vi "Panel.vi"(11 "MuxPanel in":refnum<class "MuxPanel.lvclass">) -> ()   [LabVIEW 2022 SP3, in "TouchControl.lvlib" / "MuxPanel.lvclass"]
uses:
  MuxPanel.lvclass
  C:/Program Files (x86)/National Instruments/LabVIEW 2022/vi.lib/IlluminatedG/IG OOPanel/OOPanel/Panel/Panel.lvclass
  MUX Button.ctl
  <vilib>/IlluminatedG/IG OOPanel/OOPanel/Panel/Basic UI State.ctl
  MuxPanel.lvclass/MuxPanel.ctl
  <vilib>/IlluminatedG/IG OOPanel/OOPanel/Panel/Panel.lvclass
  <vilib>/IlluminatedG/IG OOPanel/OOPanel/OOPanel.lvlib
  TouchControl.lvlib
  C:/dev/illuminatedg/TouchControl/TouchControl/MuxPanel/MuxPanel.lvclass
panel:
  in  "Desktop Bench":bool
  in  "Work Dock Bench":bool
  in  "Work Dock Main":bool
  in  "Desktop Main":bool
  in  "Input 16":bool
  in  "Input 15":bool
  in  "Input 14":bool
  in  "Input 13":bool
  in  "Input 12":bool
  in  "Input 11":bool
  in  "Input 10":bool
  in  "Input 9":bool
  in  "MUX Button 16":T1
  in  "MUX Button 15":T1
  in  "MUX Button 14":T1
  in  "MUX Button 13":T1
  in  "MUX Button 12":T1
  in  "MUX Button 11":T1
  in  "MUX Button 10":T1
  in  "MUX Button 9":T1
  in  "Input 8":bool
  in  "Input 7":bool
  in  "Input 6":bool
  in  "Input 5":bool
  in  "Input 4":bool
  in  "Input 3":bool
  in  "Input 2":bool
  in  "Input 1":bool
  in  "MUX Button 8":T1
  in  "MUX Button 7":T1
  in  "MUX Button 6":T1
  in  "MUX Button 5":T1
  in  "MUX Button 4":T1
  in  "MUX Button 3":T1
  in  "MUX Button 2":T1
  in  "MUX Button 1":T1
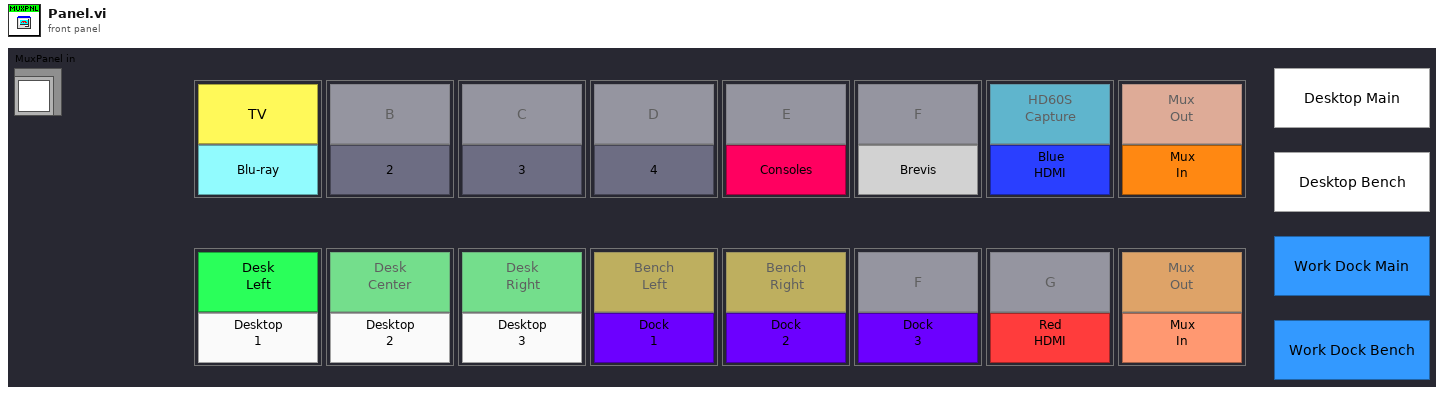
[diagram p1: front panel]
types:
  T1 = typedef "TouchControl.lvlib/MuxPanel.lvclass/MUX Button.ctl" = cluster{"A":bool, "Input":string}
  T2 = typedef "OOPanel.lvlib/Panel.lvclass/Basic UI State.ctl" = enum16{"Init", "Run", "Close"}
  T3 = typedef "TouchControl.lvlib/MUX Config.ctl" = cluster{"Outputs":T4[], "Inputs":T4[]}
  T4 = typedef "TouchControl.lvlib/MUX Element.ctl" = cluster{string, u32}
  T5 = enum8{"Enabled", "Disabled", "Disabled and Grayed Out"}
  T6 = typedef "TouchControl.lvlib/MuxPanel.lvclass/Events.ctl" = cluster{"Delay":refnum<user-event>, "Connect":refnum<user-event>}
  T7 = typedef "OOPanel.lvlib/Panel.lvclass/Panel Events.ctl" = cluster{"Visbility":refnum<user-event>, "Close":refnum<user-event>}
  T8 = typedef "TouchControl.lvlib/MUX Selection.ctl" = enum16{"Computers", "Others"}
  T9 = typedef "OOPanel.lvlib/Visibility State.ctl" = enum16{"Idle", "Closed", "Hidden", "Visible", "Subpanel", "Hidden Subpanel"}
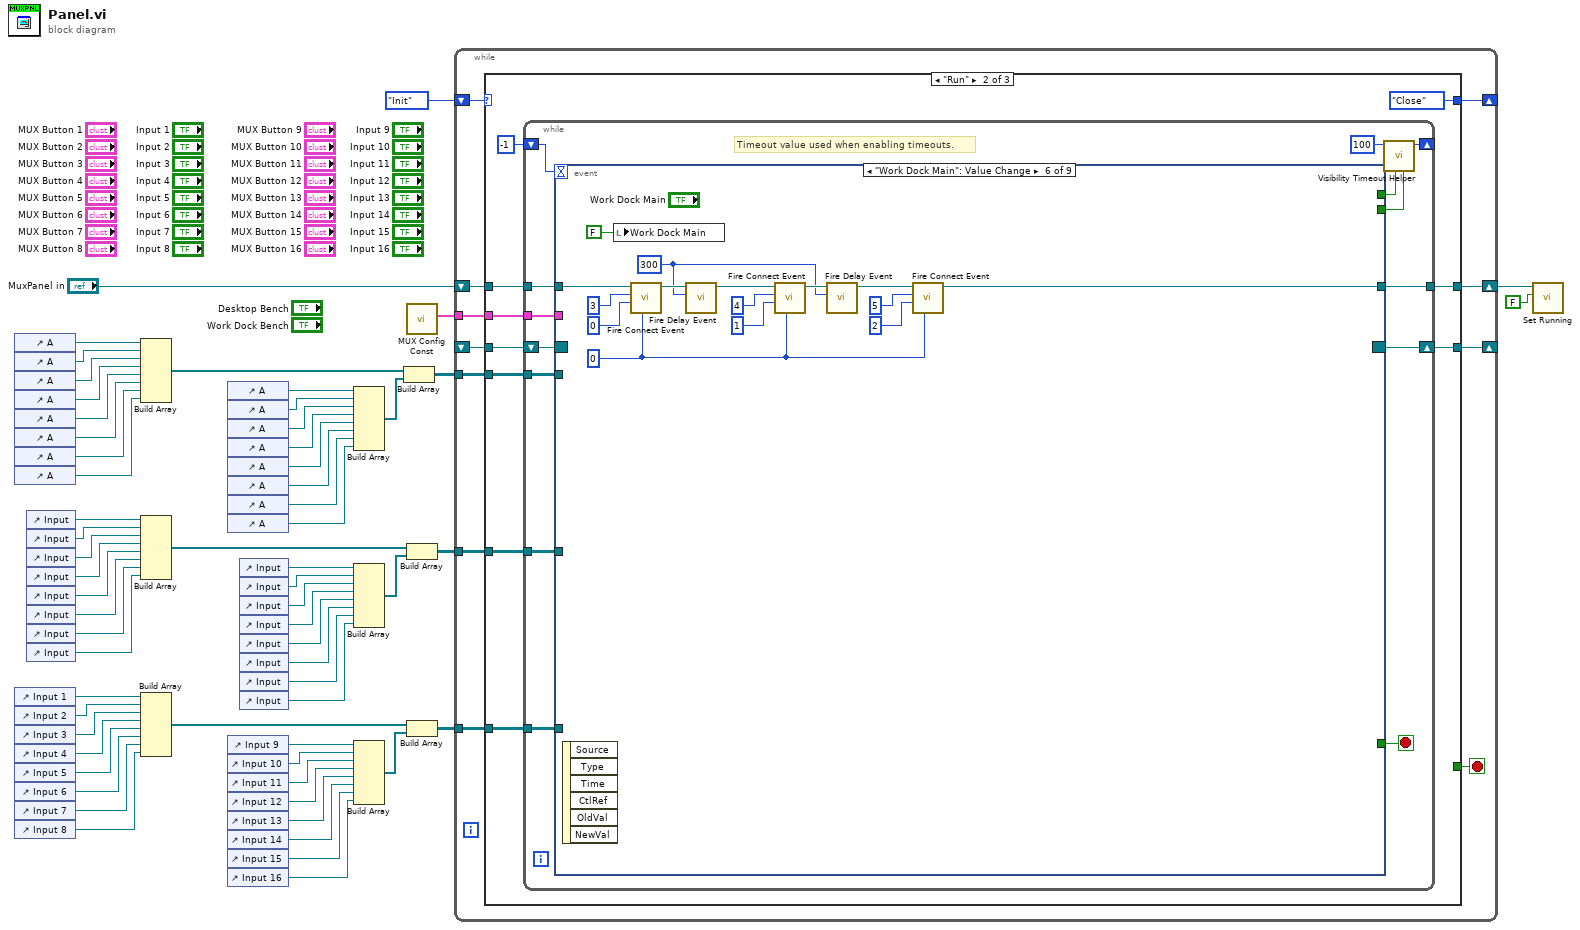
[diagram p0: block diagram]
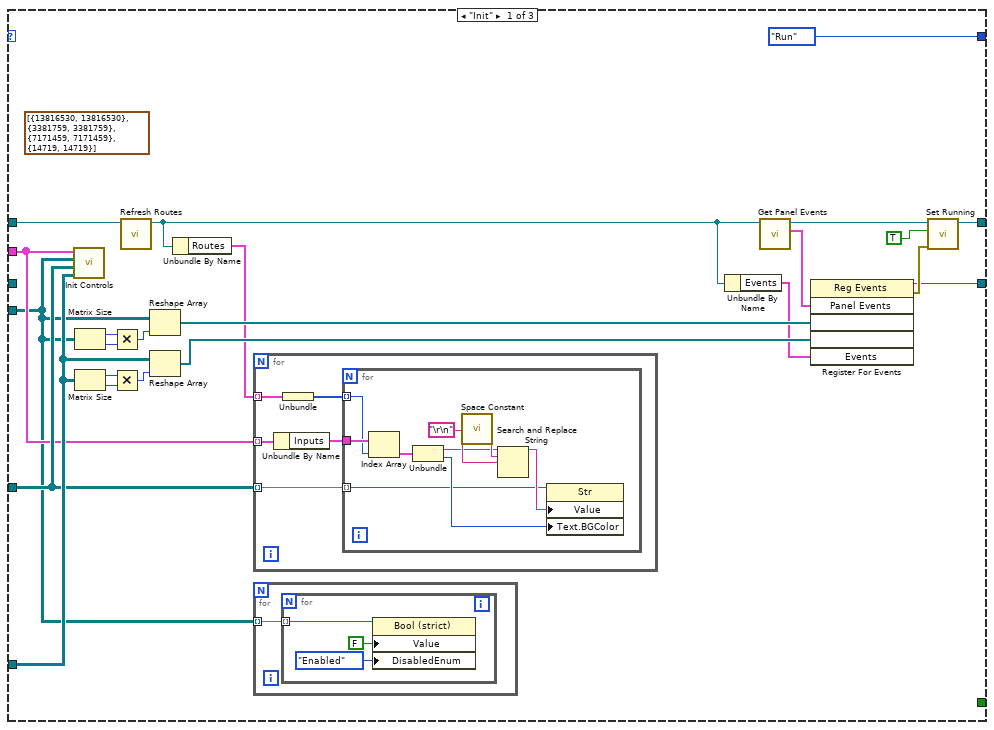
[diagram p2: hidden frame]
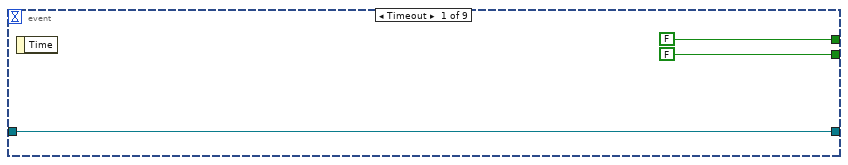
[diagram p3: hidden frame]
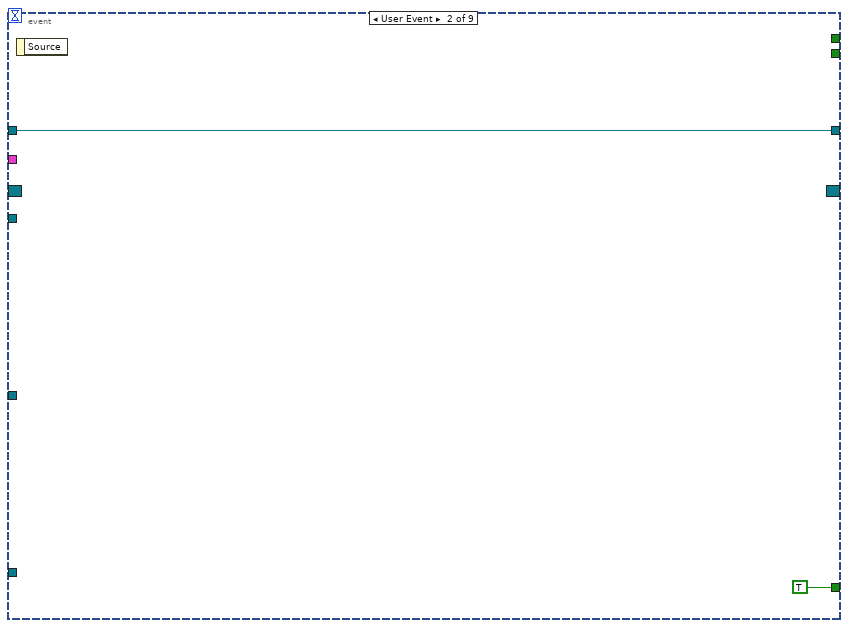
[diagram p4: hidden frame]
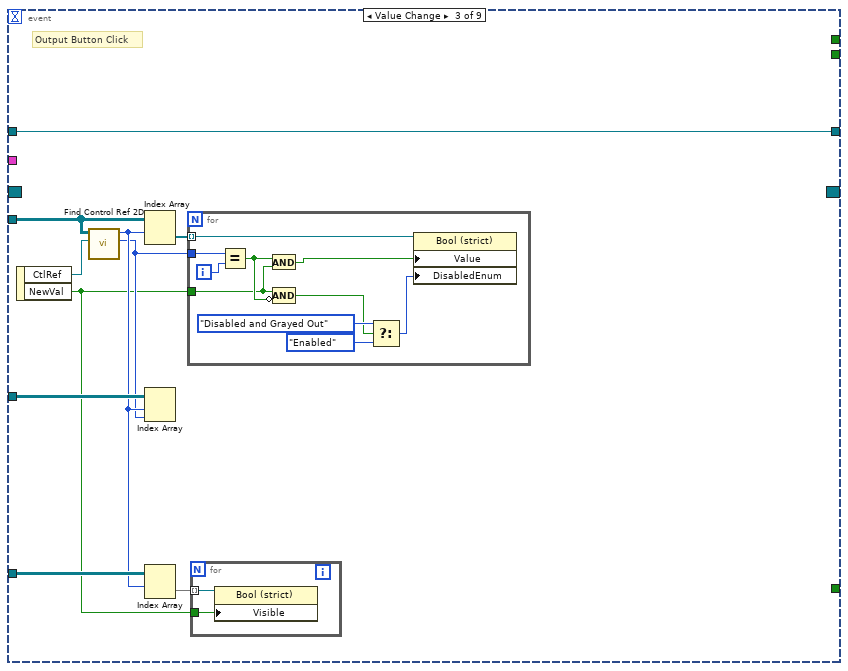
[diagram p5: hidden frame]
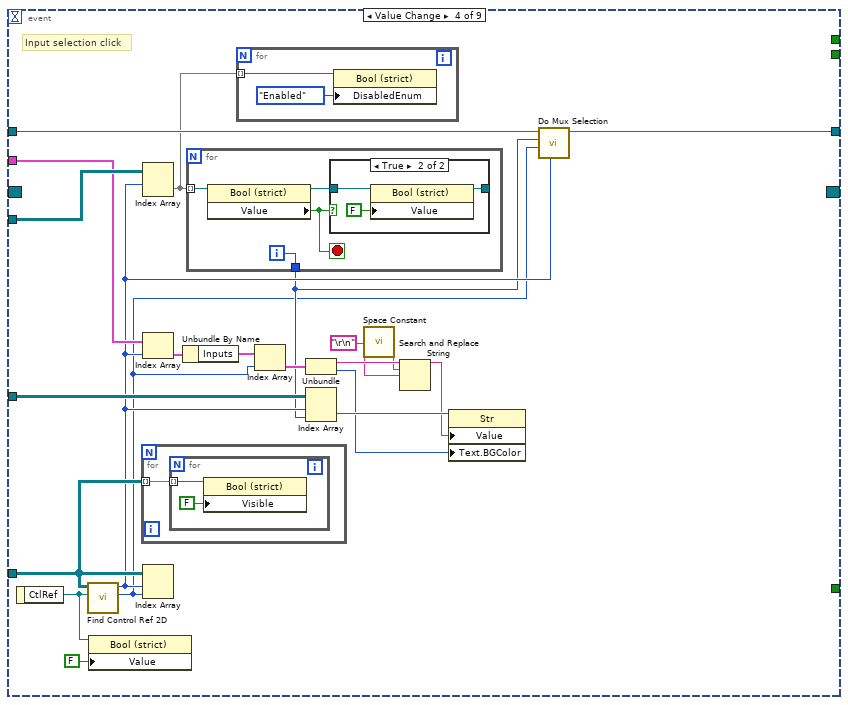
[diagram p6: hidden frame]
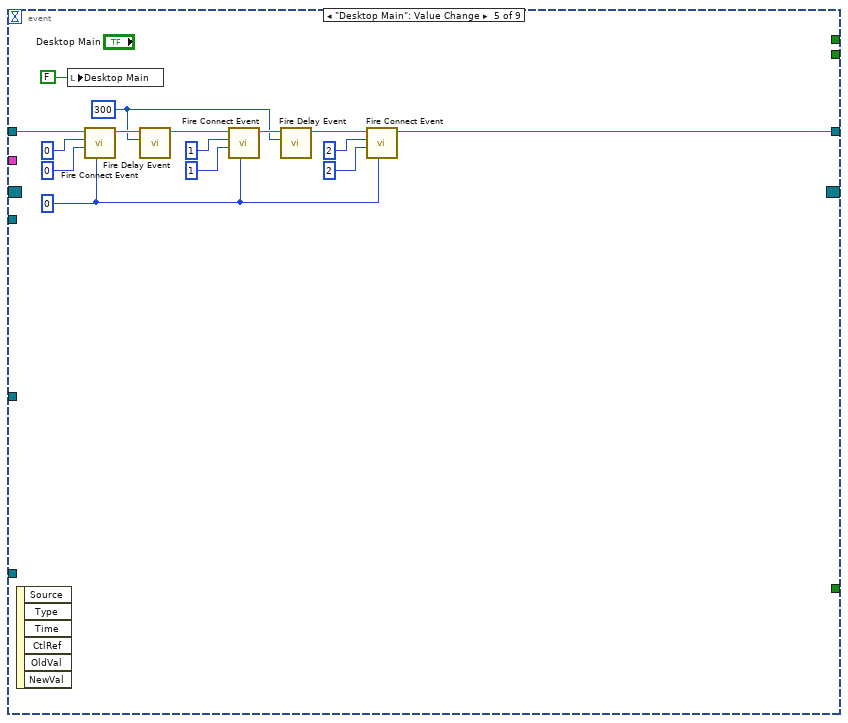
[diagram p8: hidden frame]
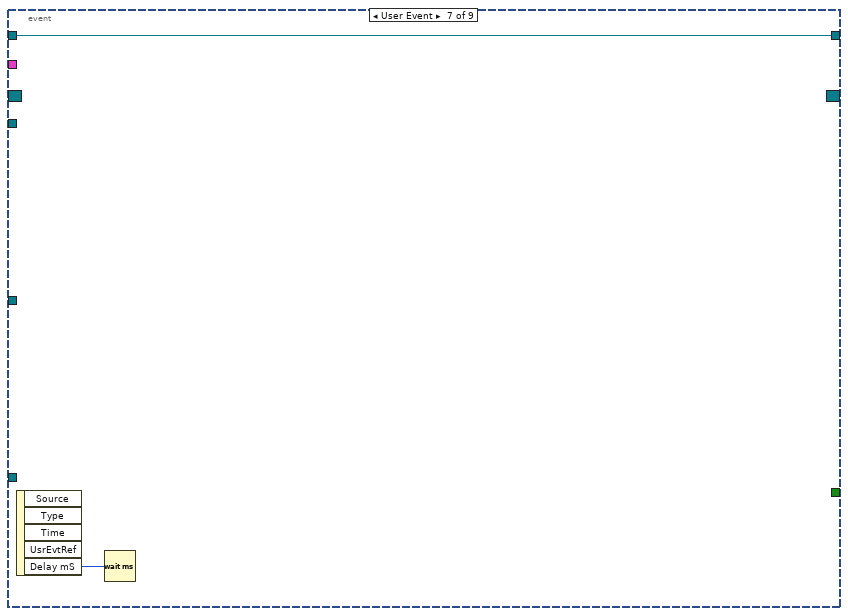
[diagram p9: hidden frame]
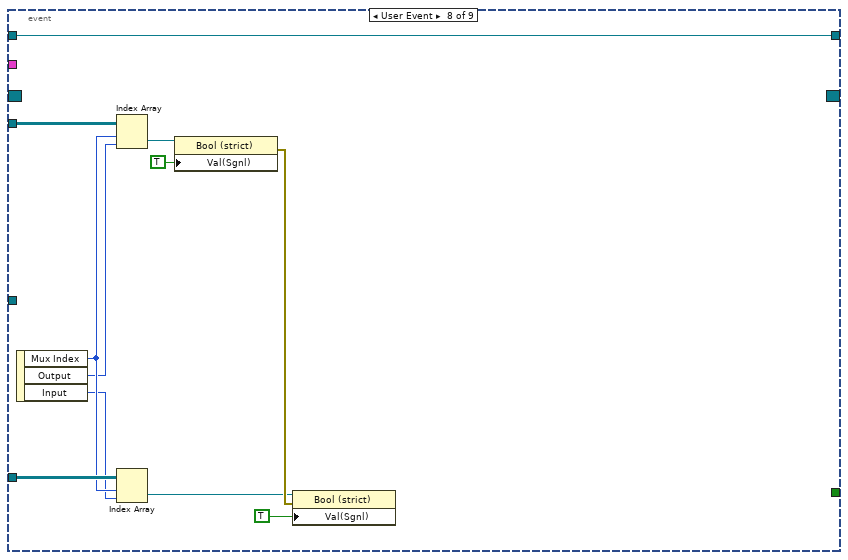
[diagram p10: hidden frame]
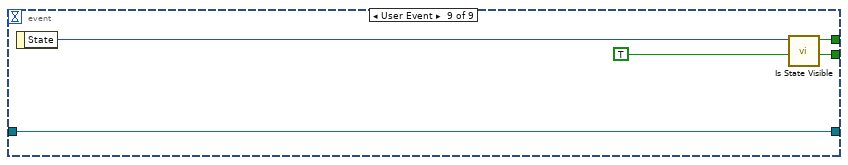
[diagram p11: hidden frame]
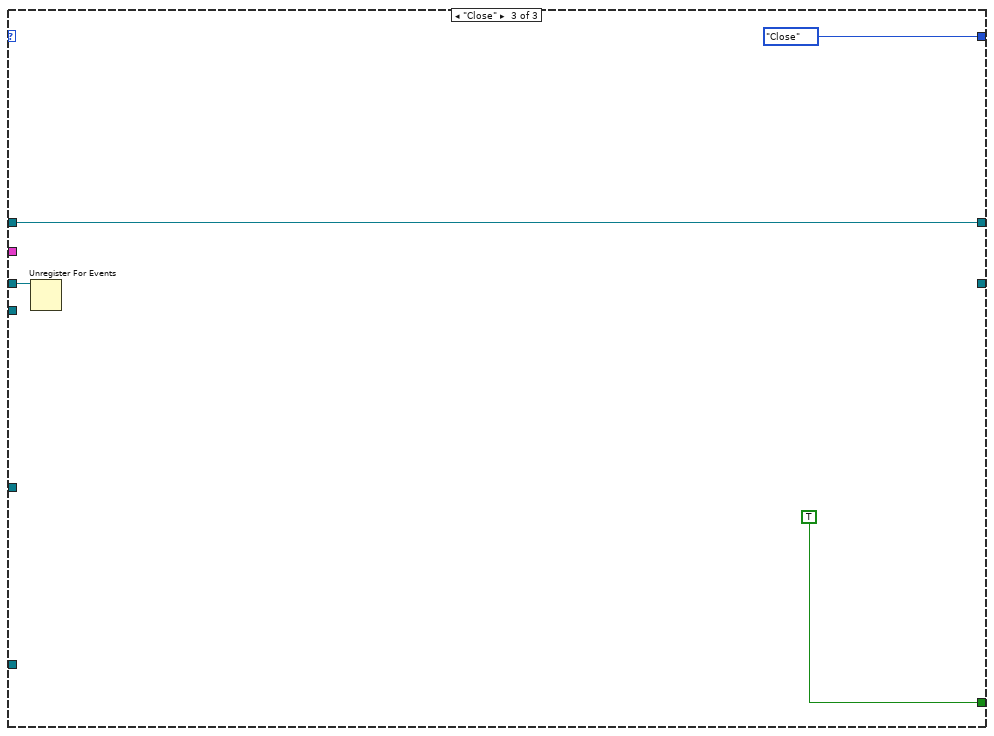
[diagram p12: hidden frame]
diagram:
  n1 = control-ref of="A"() -> (w58:refnum<vi>)
  n2 = control-ref of="A"() -> (w57:refnum<vi>)
  n3 = control-ref of="A"() -> (w56:refnum<vi>)
  n4 = control-ref of="A"() -> (w55:refnum<vi>)
  n5 = control-ref of="A"() -> (w54:refnum<vi>)
  n6 = control-ref of="A"() -> (w53:refnum<vi>)
  n7 = control-ref of="A"() -> (w52:refnum<vi>)
  n8 = control-ref of="A"() -> (w51:refnum<vi>)
  n9 = control-ref of="Input 1"() -> (w49:refnum<vi>)
  n10 = control-ref of="Input 2"() -> (w48:refnum<vi>)
  n11 = control-ref of="Input 3"() -> (w47:refnum<vi>)
  n12 = control-ref of="Input 4"() -> (w46:refnum<vi>)
  n13 = control-ref of="Input 5"() -> (w45:refnum<vi>)
  n14 = control-ref of="Input 6"() -> (w44:refnum<vi>)
  n15 = control-ref of="Input 7"() -> (w43:refnum<vi>)
  n16 = control-ref of="Input 8"() -> (w42:refnum<vi>)
  n17 = control-ref of="Input"() -> (w50:refnum<vi>)
  n18 = control-ref of="Input"() -> (w40:refnum<vi>)
  n19 = control-ref of="Input"() -> (w39:refnum<vi>)
  n20 = control-ref of="Input"() -> (w38:refnum<vi>)
  n21 = control-ref of="Input"() -> (w37:refnum<vi>)
  n22 = control-ref of="Input"() -> (w36:refnum<vi>)
  n23 = control-ref of="Input"() -> (w35:refnum<vi>)
  n24 = control-ref of="Input"() -> (w41:refnum<vi>)
  n25 = Build Array(w58, w57, w56, w55, w54, w53, w52, w51) -> (w34:refnum<vi>[])
  n26 = Build Array(w50, w40, w39, w38, w37, w36, w35, w41) -> (w33:refnum<vi>[])
  n27 = Build Array(w49, w48, w47, w46, w45, w44, w43, w42) -> (w32:refnum<vi>[])
  n28 = control-ref of="A"() -> (w8:refnum<vi>)
  n29 = control-ref of="A"() -> (w9:refnum<vi>)
  n30 = control-ref of="A"() -> (w10:refnum<vi>)
  n31 = control-ref of="A"() -> (w11:refnum<vi>)
  n32 = control-ref of="A"() -> (w12:refnum<vi>)
  n33 = control-ref of="A"() -> (w13:refnum<vi>)
  n34 = control-ref of="A"() -> (w14:refnum<vi>)
  n35 = control-ref of="A"() -> (w15:refnum<vi>)
  n36 = control-ref of="Input 9"() -> (w17:refnum<vi>)
  n37 = control-ref of="Input 10"() -> (w18:refnum<vi>)
  n38 = control-ref of="Input 11"() -> (w19:refnum<vi>)
  n39 = control-ref of="Input 12"() -> (w20:refnum<vi>)
  n40 = control-ref of="Input 13"() -> (w21:refnum<vi>)
  n41 = control-ref of="Input 14"() -> (w22:refnum<vi>)
  n42 = control-ref of="Input 15"() -> (w23:refnum<vi>)
  n43 = control-ref of="Input 16"() -> (w24:refnum<vi>)
  n44 = control-ref of="Input"() -> (w16:refnum<vi>)
  n45 = control-ref of="Input"() -> (w26:refnum<vi>)
  n46 = control-ref of="Input"() -> (w27:refnum<vi>)
  n47 = control-ref of="Input"() -> (w28:refnum<vi>)
  n48 = control-ref of="Input"() -> (w29:refnum<vi>)
  n49 = control-ref of="Input"() -> (w30:refnum<vi>)
  n50 = control-ref of="Input"() -> (w31:refnum<vi>)
  n51 = control-ref of="Input"() -> (w25:refnum<vi>)
  n52 = Build Array(w8, w9, w10, w11, w12, w13, w14, w15) -> (w6:refnum<vi>[])
  n53 = Build Array(w16, w26, w27, w28, w29, w30, w31, w25) -> (w4:refnum<vi>[])
  n54 = Build Array(w17, w18, w19, w20, w21, w22, w23, w24) -> (w2:refnum<vi>[])
  n55 = Build Array(w34, w6) -> (w7:refnum<vi>[][])
  n56 = call "MUX Config Const.vi"() -> ("MUX Config"=w1:T3[])  [unwired: 11 in]
  n57 = Build Array(w33, w4) -> (w5:refnum<vi>[][])
  n58 = Build Array(w32, w2) -> (w3:refnum<vi>[][])
  n59 = while {
    shift-right: [w72] -> _
    shift-left: _ -> [w73]
    shift-right: [w70] -> _
    shift-left: Basic_UI_State."Init" ("Basic UI State") -> [w71]
    shift-right: [w68] -> w62
    shift-left: "MuxPanel in" -> [w67]
    tunnel: w7 -> [w66]
    tunnel: w5 -> [w65]
    tunnel: w3 -> [w64]
    tunnel: w1 -> [w63]
    stop <- w69 stop-if-true
    n60 = case shown="\"Run\"" w71 {
      tunnel: w73 -> [_ w124 w248]
      tunnel: [w93 w122 _] -> w72
      tunnel: [Basic_UI_State."Run" ("Basic UI State") Basic_UI_State."Close" ("Basic UI State") Basic_UI_State."Close" ("Basic UI State")] -> w70
      tunnel: [_ _ TRUE] -> w69
      tunnel: [w92 w119 w247] -> w68
      tunnel: w67 -> [w91 w120 w247]
      tunnel: w66 -> [w74 w118 _]
      tunnel: w65 -> [w79 w117 _]
      tunnel: w64 -> [w81 w116 _]
      tunnel: w63 -> [w78 w115 _]
      frame "Init" {
        (unwired) cluster{u32, u32}[] [{13816530, 13816530}, {3381759, 3381759}, {7171459, 7171459}, {14719, 14719}] ("Colors [4]")
        n61 = call "Init Controls.vi"("Inputs"=w81, "Labels"=w79, "Outputs"=w74, "MUX Config"=w78) -> ()  [unwired: 8 in]
        n62 = Matrix Size(0:w74) -> (1:w88:i32, 2:w87:i32)
        n63 = Matrix Size(0:w81) -> (1:w84:i32, 2:w83:i32)
        n64 = Multiply(x=w88, y=w87) -> (x*y=w86:i32)
        n65 = Multiply(x=w84, y=w83) -> (x*y=w82:i32)
        n66 = call "Refresh Routes.vi"("MuxPanel in"=w91) -> ("MuxPanel out"=w76:refnum<class "MuxPanel.lvclass">)  [unwired: 9 in, 1 out]
        n67 = Reshape Array(w74, w86) -> (w85:refnum<vi>[])
        n68 = Reshape Array(w81, w82) -> (w80:refnum<vi>[])
        n69 = Unbundle By Name(w76) -> ("Routes"=w77:cluster{"Mux Route":i32[]}[])
        n70 = for {
          tunnel: w79 -> [w101] mode=indexing
          tunnel: w78 -> [w105] mode=indexing
          tunnel: w77 -> [w104] mode=indexing
          n71 = Unbundle By Name(w105) -> ("Inputs"=w102:T4[])
          n72 = Unbundle(w104) -> ("Mux Route"=w103:i32[])
          n73 = for {
            tunnel: w103 -> [w110] mode=indexing
            tunnel: w102 -> [w111]
            tunnel: w101 -> [w106] mode=indexing
            n74 = Index Array(array=w111, index=w110) -> (element=w109:T4)
            n75 = Unbundle(w109) -> (w108:string, w107:u32)
            n76 = call <vilib>:"Space Constant.vi"() -> ("String"=w114:string)
            n77 = Search and Replace String(input string=w108, search string=w114, replace string="\r\n") -> (result string=w112:string)  [unwired: 5 in, 3 out]
            n78 = property class="Str"(reference=w106, "Value"=w112, "Text.BGColor"=w107) -> ()  [unwired: 1 in, 2 out]
          }
        }
        n79 = for {
          tunnel: w74 -> [w97] mode=indexing
          n80 = for {
            tunnel: w97 -> [w100] mode=indexing
            n81 = property class="Bool (strict)"(reference=w100, "Value"=FALSE, "DisabledEnum"=T5."Enabled" ("Disabled")) -> ()  [unwired: 1 in, 2 out]
          }
        }
        n82 = Unbundle By Name(w76) -> ("Events"=w75:T6)
        n83 = call <vilib>:"Get Panel Events.vi"("Panel in"=w76) -> ("Panel Events"=w89:T7, "Panel out"=w90:refnum<class "MuxPanel.lvclass">)  [unwired: 8 in, 1 out]
        n84 = register-events(w89, w85, w80, w75) -> (reference out=w93:refnum<event-registration>, error out=w95:errorcluster)  [unwired: 2 in]
        n85 = call <vilib>:"Set Running.vi"("error in (no error)"=w95, "Running"=TRUE, "Panel in"=w90) -> ("Panel out"=w92:refnum<class "MuxPanel.lvclass">)  [unwired: 7 in, 1 out]
      }
      frame "Run" {
        n86 = while {
          shift-right: [w134] -> w122
          shift-left: w124 -> [w135]
          shift-right: [w137] -> _
          shift-left: -1 ("Timeout") -> [w136]
          tunnel: w120 -> [w130]
          tunnel: [w129] -> w119
          tunnel: w118 -> [w128]
          tunnel: w117 -> [w127]
          tunnel: w116 -> [w126]
          tunnel: w115 -> [w125]
          stop <- w131 stop-if-true
          # "Timeout value used when enabling timeouts."
          n87 = event shown="[5] \"Work Dock Main\": Value Change" {
            selector: w135 -> [_ _ _ _ _ _ _ _ _]
            dyn-events: [_ _ _ _ _ _ _ _ _] -> w134
            timeout: w136 -> [_ _ _ _ _ _ _ _ _]
            tunnel: [FALSE _ _ _ _ _ _ _ w245] -> w133
            tunnel: [FALSE _ _ _ _ _ _ _ TRUE] -> w132
            tunnel: [_ TRUE _ _ _ _ _ _ _] -> w131
            tunnel: w130 -> [w139 w142 w153 w185 w214 w229 w231 w241 w243]
            tunnel: [w139 w142 w153 w169 w200 w215 w231 w241 w243] -> w129
            tunnel: w128 -> [_ _ w151 w184 _ _ _ w240 _]
            tunnel: w127 -> [_ _ w150 w183 _ _ _ _ _]
            tunnel: w126 -> [_ _ w149 w182 _ _ _ w239 _]
            tunnel: w125 -> [_ _ _ w181 _ _ _ _ _]
            event Timeout {
              n88 = event-data() -> ()  [unwired: 1 in, 1 out]
            }
            event User Event {
              n89 = event-data() -> ()  [unwired: 1 in, 1 out]
            }
            event Value Change {
              # "Output Button Click"
              n90 = event-data() -> ("CtlRef"=w152:refnum<vi>, "NewVal"=w144:bool)  [unwired: 1 in]
              n91 = call "Find Control Ref 2D.vi"("Ctl Refnum"=w152, "2D Array"=w151) -> ("Index"=w145:i32, "MUX Selection"=w148:T8)  [unwired: 8 in]
              n92 = Index Array(array=w151, index (row)=w148) -> (element=w146:refnum<vi>[])  [unwired: 1 in]
              n93 = Index Array(array=w150, index (row)=w148, index (col)=w145) -> ()  [unwired: 1 out]
              n94 = Index Array(array=w149, index (row)=w148) -> (element=w147:refnum<vi>[])  [unwired: 1 in]
              n95 = for {
                tunnel: w146 -> [w163] mode=indexing
                tunnel: w145 -> [w162]
                tunnel: w144 -> [w155]
                i -> [w157]
                n96 = Equal?(x=w162, y=w157) -> (x = y?=w156:bool)
                n97 = And(x=w156, y=w155) -> (x .and. y?=w161:bool)
                n98 = Compound Arithmetic op=AND(w155, invert w156) -> (w154:bool)
                n99 = Select(t=T5."Disabled and Grayed Out" ("Disabled"), s=w154, f=T5."Enabled" ("Disabled")) -> (s? t:f=w158:T5)
                n100 = property class="Bool (strict)"(reference=w163, "Value"=w161, "DisabledEnum"=w158) -> ()  [unwired: 1 in, 2 out]
              }
              n101 = for {
                tunnel: w147 -> [w165] mode=indexing
                tunnel: w144 -> [w164]
                n102 = property class="Bool (strict)"(reference=w165, "Visible"=w164) -> ()  [unwired: 1 in, 2 out]
              }
            }
            event Value Change {
              # "Input selection click"
              n103 = event-data() -> ("CtlRef"=w177:refnum<vi>)  [unwired: 1 in]
              n104 = call "Find Control Ref 2D.vi"("Ctl Refnum"=w177, "2D Array"=w182) -> ("Index"=w166:i32, "MUX Selection"=w168:T8)  [unwired: 8 in]
              n105 = property class="Bool (strict)"(reference=w177, "Value"=FALSE) -> ()  [unwired: 1 in, 2 out]
              n106 = for {
                tunnel: w182 -> [w197] mode=indexing
                n107 = for {
                  tunnel: w197 -> [w199] mode=indexing
                  n108 = property class="Bool (strict)"(reference=w199, "Visible"=FALSE) -> ()  [unwired: 1 in, 2 out]
                }
              }
              n109 = Index Array(array=w184, index (row)=w168) -> (element=w170:refnum<vi>[])  [unwired: 1 in]
              n110 = Index Array(array=w181, index=w168) -> (element=w180:T3)
              n111 = Index Array(array=w182, index (row)=w168, index (col)=w166) -> ()  [unwired: 1 out]
              n112 = Unbundle By Name(w180) -> ("Inputs"=w179:T4[])
              n113 = for {
                tunnel: w170 -> [w192] mode=indexing
                tunnel: [w189] -> w167
                i -> [w189]
                stop <- w190 stop-if-true
                n114 = property class="Bool (strict)"(reference=w192) -> (reference out=w191:refnum<vi>, "Value"=w190:bool)  [unwired: 1 in, 1 out]
                n115 = case shown="True" w190 {
                  tunnel: w191 -> [w193 w196]
                  tunnel: [w193 w194] -> _
                  frame False {
                  }
                  frame True {
                    n116 = property class="Bool (strict)"(reference=w196, "Value"=FALSE) -> (reference out=w194:refnum<vi>)  [unwired: 1 in, 1 out]
                  }
                }
              }
              n117 = for {
                tunnel: w170 -> [w187] mode=indexing
                n118 = property class="Bool (strict)"(reference=w187, "DisabledEnum"=T5."Enabled" ("Disabled")) -> ()  [unwired: 1 in, 2 out]
              }
              n119 = Index Array(array=w179, index=w166) -> (element=w178:T4)
              n120 = Unbundle(w178) -> (w186:string, w174:u32)
              n121 = Index Array(array=w183, index (row)=w168, index (col)=w167) -> (element=w175:refnum<vi>)
              n122 = call <vilib>:"Space Constant.vi"() -> ("String"=w173:string)
              n123 = Search and Replace String(input string=w186, search string=w173, replace string="\r\n") -> (result string=w171:string)  [unwired: 5 in, 3 out]
              n124 = property class="Str"(reference=w175, "Value"=w171, "Text.BGColor"=w174) -> ()  [unwired: 1 in, 2 out]
              n125 = call "Do Mux Selection.vi"("MUX Selection"=w168, "Input Index"=w166, "Output Index"=w167, "MuxPanel in"=w185) -> ("MuxPanel out"=w169:refnum<class "MuxPanel.lvclass">)  [unwired: 6 in, 1 out]
            }
            event "Desktop Main": Value Change {
              w205 = 300 ("Delay mS")
              w201 = 0 ("Mux Index")
              n126 = event-data() -> ()  [unwired: 1 in, 6 out]
              n127 = local write "Desktop Main"(FALSE ("Set Desktop")) -> ()
              n128 = call "Fire Connect Event.vi"("Mux Index"=w201, "Output"=0 ("Mux Index"), "Input"=0 ("Mux Index"), "MuxPanel in"=w214) -> ("MuxPanel out"=w212:refnum<class "MuxPanel.lvclass">)  [unwired: 6 in, 1 out]
              n129 = call "Fire Delay Event.vi"("Delay mS"=w205, "MuxPanel in"=w212) -> ("MuxPanel out"=w207:refnum<class "MuxPanel.lvclass">)  [unwired: 8 in, 1 out]
              n130 = call "Fire Connect Event.vi"("Mux Index"=w201, "Output"=1 ("Mux Index"), "Input"=1 ("Mux Index"), "MuxPanel in"=w207) -> ("MuxPanel out"=w206:refnum<class "MuxPanel.lvclass">)  [unwired: 6 in, 1 out]
              n131 = call "Fire Delay Event.vi"("Delay mS"=w205, "MuxPanel in"=w206) -> ("MuxPanel out"=w202:refnum<class "MuxPanel.lvclass">)  [unwired: 8 in, 1 out]
              n132 = call "Fire Connect Event.vi"("Mux Index"=w201, "Output"=2 ("Mux Index"), "Input"=2 ("Mux Index"), "MuxPanel in"=w202) -> ("MuxPanel out"=w200:refnum<class "MuxPanel.lvclass">)  [unwired: 6 in, 1 out]
            }
            event "Work Dock Main": Value Change {
              w220 = 300 ("Delay mS")
              w216 = 0 ("Mux Index")
              n133 = event-data() -> ()  [unwired: 1 in, 6 out]
              n134 = local write "Work Dock Main"(FALSE ("Set Desktop")) -> ()
              n135 = call "Fire Connect Event.vi"("Mux Index"=w216, "Output"=0 ("Mux Index"), "Input"=3 ("Mux Index"), "MuxPanel in"=w229) -> ("MuxPanel out"=w227:refnum<class "MuxPanel.lvclass">)  [unwired: 6 in, 1 out]
              n136 = call "Fire Delay Event.vi"("Delay mS"=w220, "MuxPanel in"=w227) -> ("MuxPanel out"=w222:refnum<class "MuxPanel.lvclass">)  [unwired: 8 in, 1 out]
              n137 = call "Fire Connect Event.vi"("Mux Index"=w216, "Output"=1 ("Mux Index"), "Input"=4 ("Mux Index"), "MuxPanel in"=w222) -> ("MuxPanel out"=w221:refnum<class "MuxPanel.lvclass">)  [unwired: 6 in, 1 out]
              n138 = call "Fire Delay Event.vi"("Delay mS"=w220, "MuxPanel in"=w221) -> ("MuxPanel out"=w217:refnum<class "MuxPanel.lvclass">)  [unwired: 8 in, 1 out]
              n139 = call "Fire Connect Event.vi"("Mux Index"=w216, "Output"=2 ("Mux Index"), "Input"=5 ("Mux Index"), "MuxPanel in"=w217) -> ("MuxPanel out"=w215:refnum<class "MuxPanel.lvclass">)  [unwired: 6 in, 1 out]
            }
            event User Event {
              n140 = event-data() -> ("Delay mS"=w230:i32)  [unwired: 1 in, 4 out]
              n141 = Wait (ms)(milliseconds to wait=w230) -> ()  [unwired: 1 out]
            }
            event User Event {
              n142 = event-data() -> ("Mux Index"=w238:i32, "Output"=w237:i32, "Input"=w232:i32)  [unwired: 1 in]
              n143 = Index Array(array=w240, index (row)=w238, index (col)=w237) -> (element=w236:refnum<vi>)
              n144 = Index Array(array=w239, index (row)=w238, index (col)=w232) -> (element=w234:refnum<vi>)
              n145 = property class="Bool (strict)"(reference=w236, "Val(Sgnl)"=TRUE ("Value (Signaling)")) -> (error out=w242:errorcluster)  [unwired: 1 in, 1 out]
              n146 = property class="Bool (strict)"(reference=w234, error in=w242, "Val(Sgnl)"=TRUE ("Value (Signaling)")) -> ()  [unwired: 2 out]
            }
            event User Event {
              n147 = event-data() -> ("State"=w246:T9)  [unwired: 1 in]
              n148 = call <vilib>:"Is State Visible.vi"("Visibility"=w246) -> ("Visible"=w245:bool)  [unwired: 10 in]
            }
          }
          n149 = call <vilib>:"Visibility Timeout Helper.vi"("Update?"=w132, "Use Timeout?"=w133, "Visible Timeout mS"=100) -> ("Timeout"=w137:i32)  [unwired: 8 in]
        }
      }
      frame "Close" {
        n150 = Unregister For Events(event registration refnum=w248) -> ()  [unwired: 1 in, 1 out]
      }
    }
  }
  n151 = call <vilib>:"Set Running.vi"("Running"=FALSE, "Panel in"=w62) -> ()  [unwired: 8 in, 2 out]
